vi "Max and Min 50 Batch.vi"() -> ()   [LabVIEW 2012]
panel:
  out "Batch Number":dbl
  out "Max Value":dbl
  out "Min Value":dbl
  in  "Production Rate Knob ms":dbl(knob) scale=10.0..500.0
  in  "stop":bool
  out "Max Value Waveform Chart":dbl(graph)
  out "Min Vaue Waveform Chart":dbl(graph)
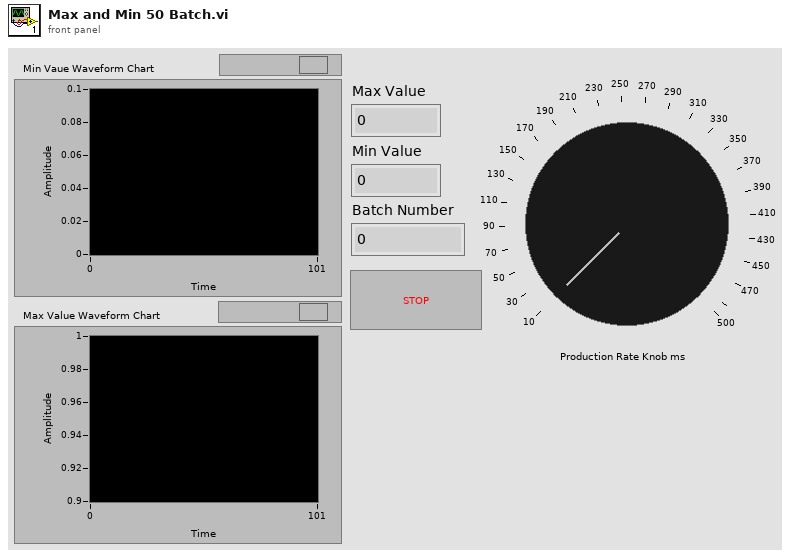
[diagram p1: front panel]
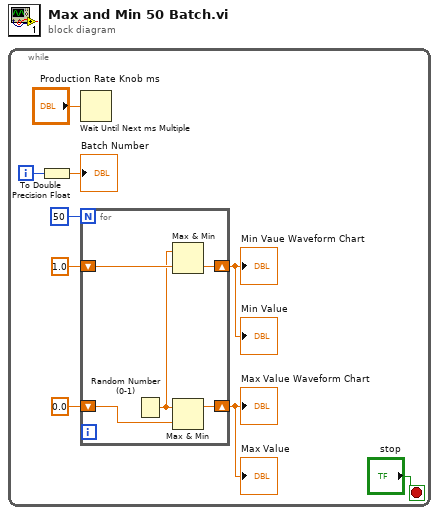
[diagram p0: block diagram]
diagram:
  n1 = while {
    i -> [w1]
    stop <- "stop" stop-if-true
    n2 = To Double Precision Float(number=w1) -> (double precision float=→"Batch Number":dbl)
    n3 = Wait Until Next ms Multiple(millisecond multiple="Production Rate Knob ms") -> ()  [unwired: 1 out]
    n4 = for {
      N: 50 -> [_]
      shift-right: [w14] -> w4
      shift-left: 1.0 -> [w13]
      shift-right: [w11] -> w3
      shift-left: 0.0 -> [w10]
      n5 = Random Number (0-1)() -> (number: 0 to 1=w12:dbl)
      n6 = Max & Min(x=w12, y=w13) -> (min(x,y)=w14:dbl)  [unwired: 1 out]
      n7 = Max & Min(x=w12, y=w10) -> (max(x,y)=w11:dbl)  [unwired: 1 out]
    }
    "Min Vaue Waveform Chart" <- w4
    "Max Value Waveform Chart" <- w3
    "Min Value" <- w4
    "Max Value" <- w3
  }
